vi "Update RPC Template Accessors.vi"(8 "error in (no error)":errorcluster, 11 "Server Library (Library Item) in":refnum<vi>) -> (0 "error out":errorcluster, 3 "Server Library (Library Item) out":refnum<vi>)   [LabVIEW 2019, in "gRPC Scripting Tools.lvlib"]
uses:
  gRPC Scripting Tools.lvlib
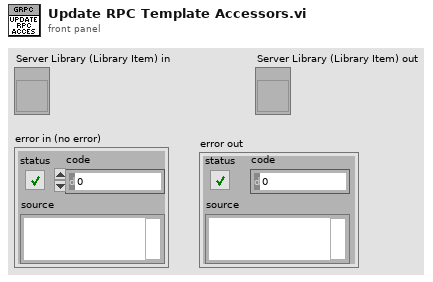
[diagram p1: front panel]
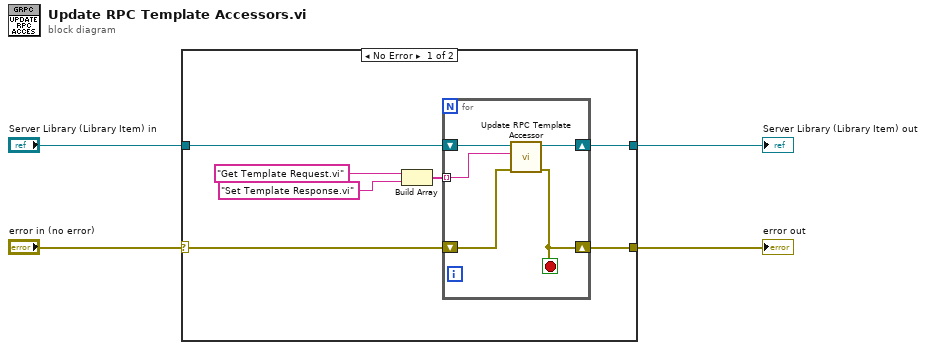
[diagram p0: block diagram]
diagram:
  n1 = case shown="No Error" "error in (no error)" {
    selector: "error in (no error)" -> [w6 w18]
    tunnel: "Server Library (Library Item) in" -> [w10 w17]
    tunnel: [w5 w18] -> w3
    tunnel: [w11 w17] -> w1
    frame No Error {
      n2 = Build Array("Get Template Request.vi" ("Item Name"), "Set Template Response.vi" ("Item Name")) -> (w7:string[])
      n3 = for {
        shift-right: [w16] -> w11
        shift-left: w10 -> [w15]
        tunnel: w7 -> [w14] mode=indexing
        shift-right: [w12] -> w5
        shift-left: w6 -> [w13]
        stop <- w12 stop-if-true
        n4 = call "Update RPC Template Accessor.vi"("error in (no error)"=w13, "Accessor Name"=w14, "Server Library (Library Item) in"=w15) -> ("error out"=w12:errorcluster, "Server Library (Library Item) out"=w16:refnum<vi>)  [unwired: 7 in]
      }
    }
    frame Error {
    }
  }
  "error out" <- w3
  "Server Library (Library Item) out" <- w1
